vi "Database.Main-Setup.vi"(8 "error in":errorcluster) -> (0 "error out":errorcluster)   [LabVIEW 2016]
uses:
  Database.Main.Action.ctl
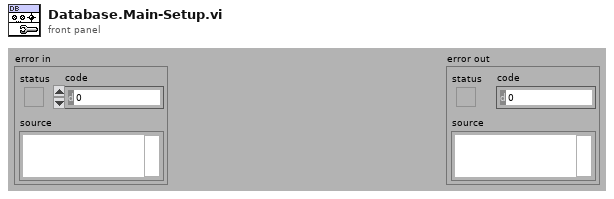
[diagram p1: front panel]
types:
  T1 = typedef "Database.Main.Action.ctl" = enum32{"idle", "constructor", "destructor", "--- DB ---", "Init", "Setup", "Select.Variant", "File.Export", "UpdateVariantFiles"}
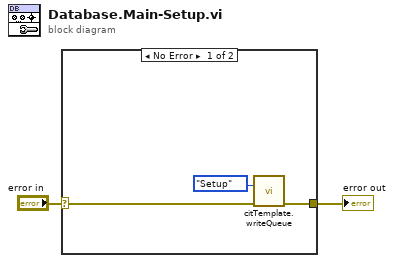
[diagram p0: block diagram]
diagram:
  n1 = case shown="No Error" "error in" {
    selector: "error in" -> [w4 w6]
    tunnel: [w5 w6] -> w1
    frame No Error {
      n2 = call "citTemplate.writeQueue.vi"("event in (if not connected:all statemachine with data event)"=Database.Main.Action."Setup" ("Action"), "error in (no error)"=w4) -> ("error out"=w5:errorcluster)  [unwired: 13 in]
    }
    frame Error {
    }
  }
  "error out" <- w1
